vi "InputDICOMVariables.vi"(7 "values":string[](array[string]), 9 "Operator":string, 10 "CPR Number":string, 11 "Name":string) -> (3 "Array":string[](array[string]))   [LabVIEW 2013, in "main.lvlib"]
uses:
  main.lvlib
panel:
  in  "keywords":string[](array[string])
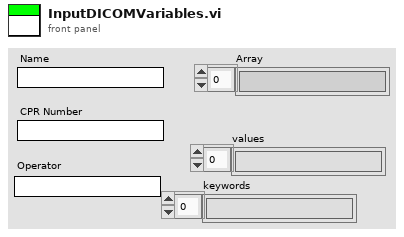
[diagram p1: front panel]
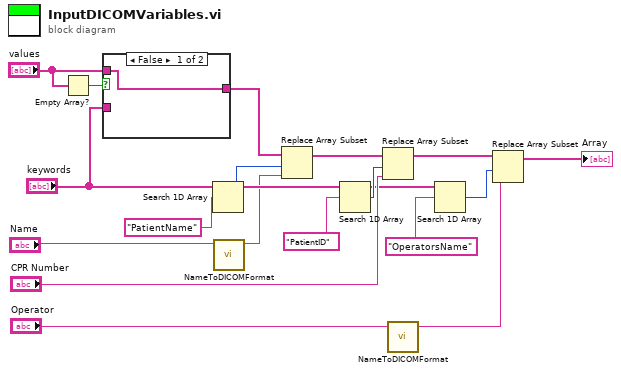
[diagram p0: block diagram]
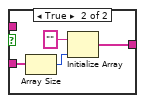
[diagram p2: hidden frame]
diagram:
  n1 = Empty Array?(array="values") -> (empty?=w7:bool)
  n2 = case shown="False" w7 {
    tunnel: "keywords" -> [_ w23]
    tunnel: [w19 w20] -> w8
    tunnel: "values" -> [w19 _]
    frame False {
    }
    frame True {
      n3 = Array Size(array=w23) -> (size(s)=w22:i32)
      n4 = Initialize Array("", w22) -> (w20:string[])
    }
  }
  n5 = Search 1D Array(1D array="keywords", element="PatientName") -> (index of element=w15:i32)  [unwired: 1 in]
  n6 = call "NameToDICOMFormat.vi"("Name In"="Name") -> ("Name Out"=w4:string)  [unwired: 10 in]
  n7 = Replace Array Subset(array=w8, new element=w4, index=w15) -> (w16:string[])
  n8 = Search 1D Array(1D array="keywords", element="PatientID") -> (index of element=w17:i32)  [unwired: 1 in]
  n9 = Replace Array Subset(array=w16, new element="CPR Number", index=w17) -> (w12:string[])
  n10 = call "NameToDICOMFormat.vi"("Name In"="Operator") -> ("Name Out"=w1:string)  [unwired: 10 in]
  n11 = Search 1D Array(1D array="keywords", element="OperatorsName") -> (index of element=w11:i32)  [unwired: 1 in]
  n12 = Replace Array Subset(array=w12, new element=w1, index=w11) -> (→"Array":string[])
